vi "Item to String.vi"(11 "Item in":T1) -> (2 "0 String":string, 3 "Item out":T1)   [LabVIEW 2015, in "Read-Write-Signals.xnode"]
uses:
  Read-Write-Signals.xnode
  Read-Write-Signals Item.ctl
  Read-Write-Signals Sub Item.ctl
  Read-Write-Signals Sub Item Type.ctl
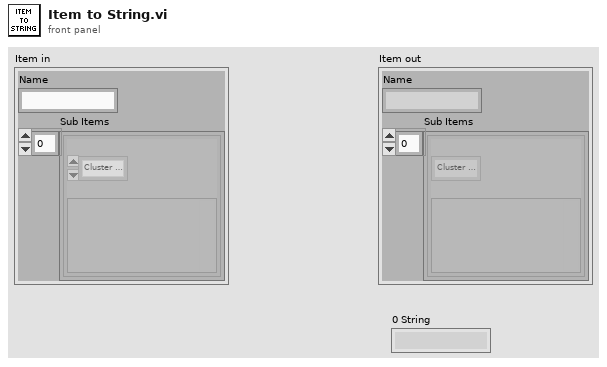
[diagram p1: front panel]
types:
  T1 = typedef "Read-Write-Signals Item.ctl" = cluster{"Name":string, "Sub Items":T2[]}
  T2 = typedef "Read-Write-Signals Sub Item.ctl" = cluster{"Type":T3, "Value":variant}
  T3 = typedef "Read-Write-Signals Sub Item Type.ctl" = enum8{"Cluster Element", "Array Element", "Subarray"}
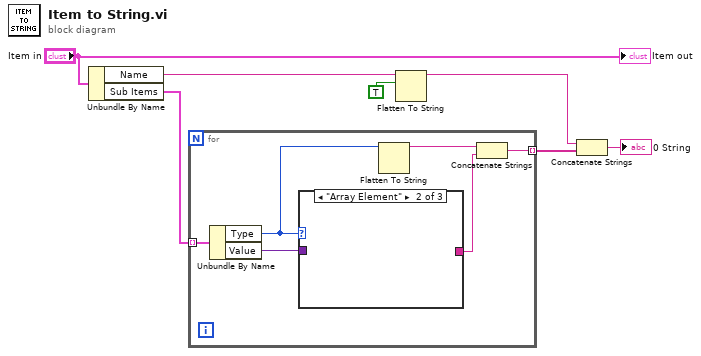
[diagram p0: block diagram]
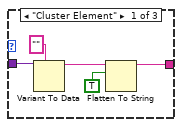
[diagram p2: hidden frame]
diagram:
  n1 = Unbundle By Name("Item in") -> ("Name"=w2:string, "Sub Items"=w3:T2[])
  n2 = for {
    tunnel: w3 -> [w13] mode=indexing
    tunnel: [w8] -> w6 mode=indexing
    n3 = Unbundle By Name(w13) -> ("Type"=w11:T3, "Value"=w12:variant)
    n4 = case shown="\"Array Element\"" w11 {
      tunnel: w12 -> [w18 _ _]
      tunnel: [w15 _ _] -> w9
      frame "Cluster Element" {
        n5 = Variant To Data(type="", Variant=w18) -> (data=w14:string)  [unwired: 1 in, 1 out]
        n6 = Flatten To String(anything=w14, prepend array or string size? (T)=TRUE) -> (data string=w15:string)  [unwired: 2 in, 2 out]
      }
      frame "Array Element" {
      }
      frame "Subarray" {
      }
    }
    n7 = Flatten To String(anything=w11) -> (data string=w10:string)  [unwired: 3 in, 2 out]
    n8 = Concatenate Strings(w10, w9) -> (w8:string)
  }
  n9 = Flatten To String(anything=w2, prepend array or string size? (T)=TRUE) -> (data string=w5:string)  [unwired: 2 in, 2 out]
  n10 = Concatenate Strings(w5, w6) -> (→"0 String":string)
  "Item out" <- "Item in"
